vi "arduinoSetValvePuffed.vi"(7 "valve data puffed":bool[](array[boolean])=[TRUE, FALSE, FALSE, FALSE, FALSE, FALSE, FALSE, FALSE], 8 "valve data close":bool[](array[boolean])=[FALSE, FALSE, FALSE, FALSE, FALSE, FALSE, FALSE, FALSE], 9 "valve data open":bool[](array[boolean])=[TRUE, FALSE, FALSE, FALSE, FALSE, FALSE, FALSE, FALSE], 10 "milliseconds to wait":u32=100, 11 "numPuffs":i32) -> ()   [LabVIEW 2012]
uses:
  GlobalValves.vi
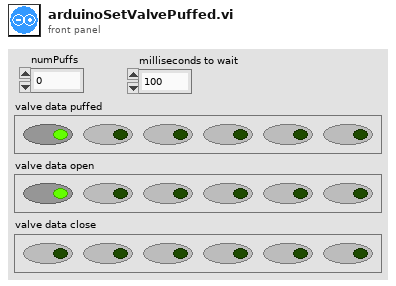
[diagram p1: front panel]
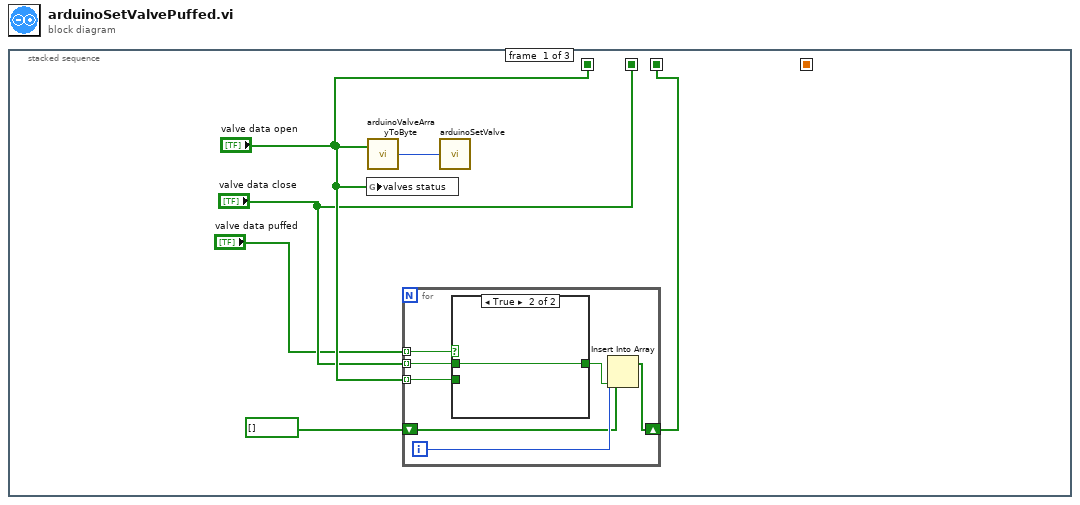
[diagram p0: block diagram]
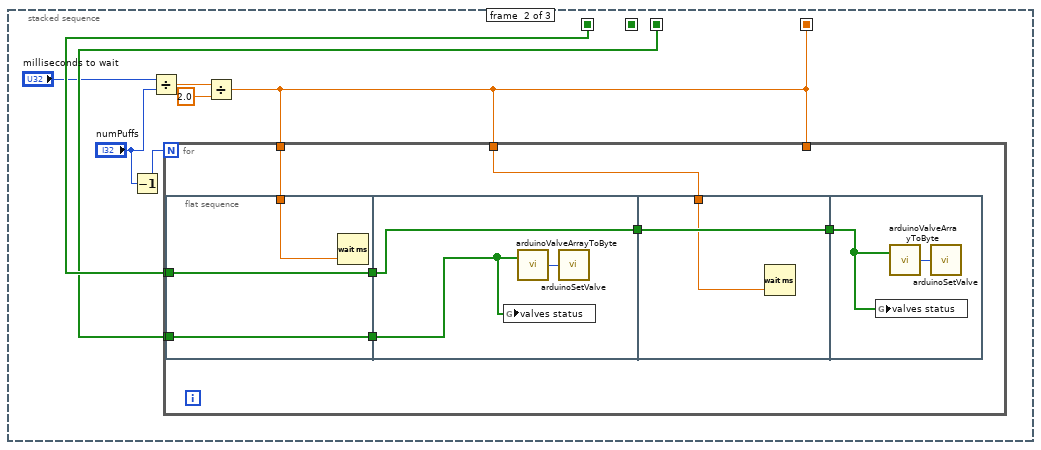
[diagram p3: hidden frame]
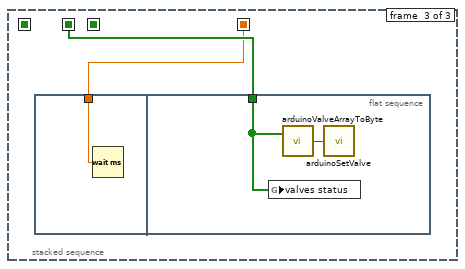
[diagram p4: hidden frame]
diagram:
  n1 = stacked-sequence {
    seq-local: ["valve data open" _ _] -> [_ w21 _]
    seq-local: ["valve data close" _ _] -> [_ _ w43]
    seq-local: [w4 _ _] -> [_ w20 _]
    seq-local: [_ w19 _] -> [_ _ w42]
    frame #0 {
      n2 = global write "GlobalValves.vi" "valves status"("valve data open") -> ()
      n3 = call "arduinoValveArrayToByte.vi"("valve data open"="valve data open") -> ("output"=w1:u8)  [unwired: 1 in]
      n4 = for {
        tunnel: "valve data close" -> [w12] mode=indexing
        tunnel: "valve data puffed" -> [w13] mode=indexing
        tunnel: "valve data open" -> [w11] mode=indexing
        shift-right: [w7] -> w4
        shift-left: bool[] [] ("array") -> [w8]
        i -> [w9]
        n5 = case shown="True" w13 {
          tunnel: w12 -> [_ w15]
          tunnel: [w14 w15] -> w10
          tunnel: w11 -> [w14 _]
          frame False {
          }
          frame True {
          }
        }
        n6 = Insert Into Array(array=w8, index=w9, new element=w10) -> (w7:bool[])
      }
      n7 = call "arduinoSetValve.vi"("command"=w1) -> ()
    }
    frame #1 {
      n8 = Decrement(x="numPuffs") -> (x-1=w16:i32)
      n9 = Divide(x="milliseconds to wait", y="numPuffs") -> (x/y=w22:dbl)
      n10 = Divide(x=w22, y=2.0) -> (x/y=w19:dbl)
      n11 = for {
        N: w16 -> [_]
        tunnel: w21 -> [w31]
        tunnel: w20 -> [w30]
        tunnel: w19 -> [w27]
        tunnel: w19 -> [_]
        tunnel: w19 -> [w24]
        n12 = flat-sequence {
          tunnel: w30 -> [w33]
          tunnel: w31 -> [w34]
          tunnel: [w34] -> w26
          tunnel: [w33] -> w25
          tunnel: w24 -> [w32]
          tunnel: [w35] -> w28
          tunnel: w26 -> [w35]
          tunnel: w25 -> [w36]
          tunnel: [w39] -> w29
          tunnel: w28 -> [w39]
          tunnel: w27 -> [w38]
          tunnel: w29 -> [w40]
          frame #0 {
            n13 = Wait (ms)(milliseconds to wait=w32) -> ()  [unwired: 1 out]
          }
          frame #1 {
            n14 = global write "GlobalValves.vi" "valves status"(w36) -> ()
            n15 = call "arduinoValveArrayToByte.vi"("valve data open"=w36) -> ("output"=w37:u8)  [unwired: 1 in]
            n16 = call "arduinoSetValve.vi"("command"=w37) -> ()
          }
          frame #2 {
            n17 = Wait (ms)(milliseconds to wait=w38) -> ()  [unwired: 1 out]
          }
          frame #3 {
            n18 = global write "GlobalValves.vi" "valves status"(w40) -> ()
            n19 = call "arduinoValveArrayToByte.vi"("valve data open"=w40) -> ("output"=w41:u8)  [unwired: 1 in]
            n20 = call "arduinoSetValve.vi"("command"=w41) -> ()
          }
        }
      }
    }
    frame #2 {
      n21 = flat-sequence {
        tunnel: w42 -> [w44]
        tunnel: w43 -> [w45]
        frame #0 {
          n22 = Wait (ms)(milliseconds to wait=w44) -> ()  [unwired: 1 out]
        }
        frame #1 {
          n23 = global write "GlobalValves.vi" "valves status"(w45) -> ()
          n24 = call "arduinoValveArrayToByte.vi"("valve data open"=w45) -> ("output"=w46:u8)  [unwired: 1 in]
          n25 = call "arduinoSetValve.vi"("command"=w46) -> ()
        }
      }
    }
  }
